vi "Stall A arm Lower.vi"(7 "Port (Port A)":T1 items=["Port A", "Port B", "Port C", "Port D"], 9 "Power":i8=30, 11 "NXT/EV3":T2) -> (3 "NXT/EV3":T2)   [LabVIEW 2015]
uses:
  <vilib>/NXT/Block Support/NXT_TimerIndex.ctl
  <vilib>/NXT/Block Support/NXT_OutputPort.ctl
  <vilib>/NXT/Dual Mode Library/Motors/Rotation.vi
  <vilib>/NXT/Dual Mode Library/Sensors/Reset_Timer.vi
  <vilib>/NXT/Dual Mode Library/Waits/Wait_Num.vi
  <vilib>/NXT/LegoClasses/BrickReference/BrickReference.lvclass
  <vilib>/NXT/Subs/LVHSConnector.ctl
  <vilib>/NXT/NXTIO Xnodes/NXTIOXNode/NXTIO.xnode
  <vilib>/NXT/Dual Mode Library/Sensors/Read_Timer.vi
  <vilib>/NXT/NXTIO Xnodes/NXTIONodeSubVIs/NXTMoveMotors.vi
  <vilib>/NXT/NXTIO Xnodes/NXTIONodeSubVIs/LEGOResetMotors.vi
  <vilib>/NXT/NXTIO Xnodes/NXTIONodeSubVIs/NXTStopMotors.vi
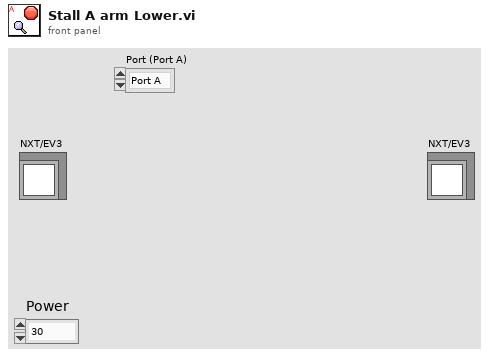
[diagram p1: front panel]
types:
  T1 = typedef "NXT_OutputPort.ctl" = u8
  T2 = typedef "LVHSConnector.ctl" = refnum<class "BrickReference.lvclass">
  T3 = typedef "NXT_TimerIndex.ctl" = u8
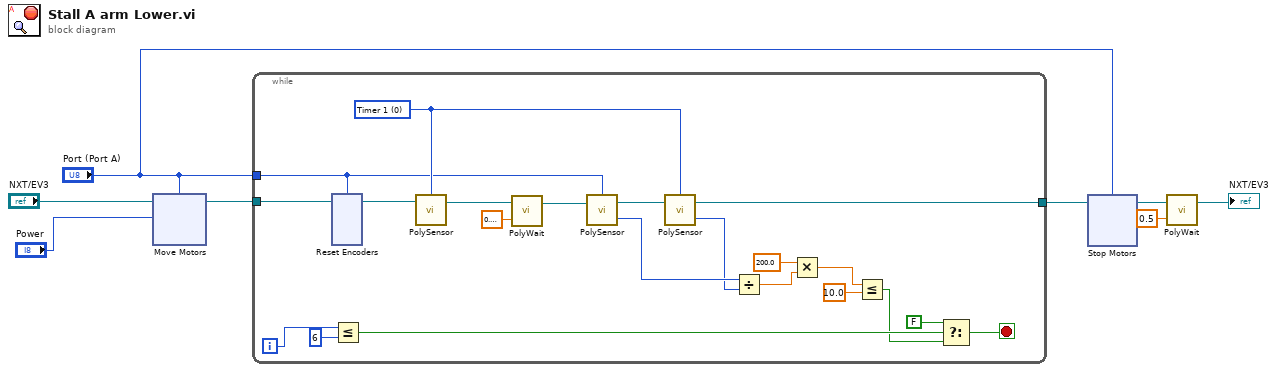
[diagram p0: block diagram]
diagram:
  n1 = xnode "Move Motors"("Power/Speed 1"="Power", "Motors"="Port (Port A)", "NXT/EV3"="NXT/EV3") -> ("NXT/EV3"=w8:T2)
  n2 = while {
    tunnel: w8 -> [w21]
    tunnel: [w20] -> w7
    tunnel: "Port (Port A)" -> [w19]
    i -> [w10]
    stop <- w13 stop-if-true
    w25 = T3 0 items=["Timer 1", "Timer 2", "Timer 3"] ("Timer (Timer 1)")
    n3 = xnode "Reset Encoders"("Motors"=w19, "NXT/EV3"=w21) -> ("NXT/EV3"=w29:T2)
    n4 = Less Or Equal?(x=w10, y=6) -> (x <= y?=w15:bool)
    n5 = call-poly <vilib>:"PolySensor.vi"("NXT/EV3"=w29, "Timer (Timer 1)"=w25) -> ("NXT/EV3"=w28:T2)  [unwired: 2 in]
    n6 = call-poly <vilib>:"PolyWait.vi"("Time (1 sec)"=sgl 0.1, "NXT/EV3"=w28) -> ("NXT/EV3"=w26:T2)  [unwired: 2 in]
    n7 = call-poly <vilib>:"PolySensor.vi"("NXT/EV3"=w26, "Port (Port A)"=w19) -> ("Angle of Rotation"=w23:i32, "NXT/EV3"=w24:T2)  [unwired: 1 in]
    n8 = call-poly <vilib>:"PolySensor.vi"("NXT/EV3"=w24, "Timer (Timer 1)"=w25) -> ("Value (msec)"=w22:u32, "NXT/EV3"=w20:T2)  [unwired: 1 in]
    n9 = Divide(x=w23, y=w22) -> (x/y=w18:dbl)
    n10 = Multiply(x=200.0, y=w18) -> (x*y=w17:dbl)
    n11 = Less Or Equal?(x=w17, y=10.0) -> (x <= y?=w12:bool)
    n12 = Select(t=FALSE, s=w15, f=w12) -> (s? t:f=w13:bool)
  }
  n13 = xnode "Stop Motors"("Motors"="Port (Port A)", "NXT/EV3"=w7) -> ("NXT/EV3"=w4:T2)
  n14 = call-poly <vilib>:"PolyWait.vi"("Time (1 sec)"=sgl 0.5, "NXT/EV3"=w4) -> ("NXT/EV3"=→"NXT/EV3":T2)  [unwired: 2 in]
